vi "Parsing Error (inlined).vi"(7 "JSON":string, 8 "error in (no error)":errorcluster, 9 "Offset past match":i32=-1, 10 "Value start":i32=-1, 11 "State":T1) -> (0 "error out":errorcluster, 3 "Value (if no error)":string)   [LabVIEW 2019, in "JSONtext.lvlib"]
uses:
  JSONtext.lvlib
  Parsing State.ctl
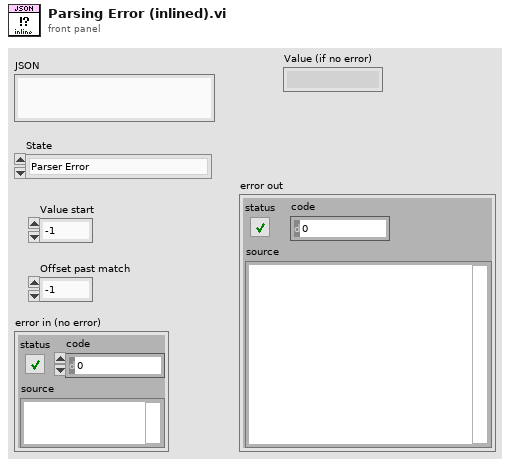
[diagram p1: front panel]
types:
  T1 = typedef "JSONtext.lvlib/Parsing State.ctl" = enum16{"Parser Error", "Object", "Array", "String", "Number/Other", "Leading Whitespace", "Object end", "Array end", "Value end"}
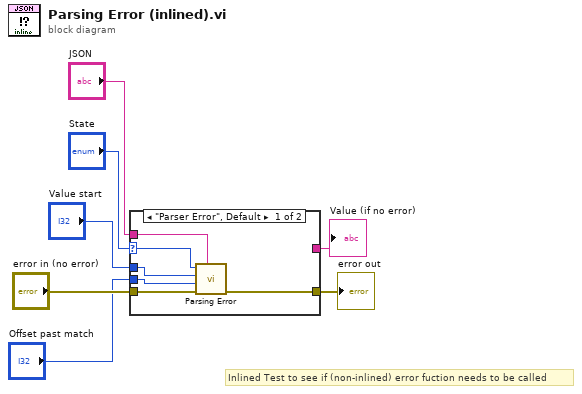
[diagram p0: block diagram]
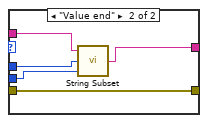
[diagram p2: hidden frame]
diagram:
  # "Inlined Test to see if (non-inlined) error fuction needs to be called"
  n1 = case shown="\"Parser Error\", Default" "State" {
    selector: "State" -> [w8 _]
    tunnel: "JSON" -> [w13 w17]
    tunnel: "error in (no error)" -> [w12 w18]
    tunnel: [w11 w18] -> w6
    tunnel: "Value start" -> [w10 w16]
    tunnel: "Offset past match" -> [w9 w15]
    tunnel: [_ w14] -> w1
    frame "Parser Error", Default {
      n2 = call "Parsing Error.vi"("JSON"=w13, "error in (no error)"=w12, "Offset past match"=w9, "Value start"=w10, "State"=w8) -> ("error out"=w11:errorcluster)  [unwired: 6 in]
    }
    frame "Value end" {
      n3 = call "String Subset.vi"("Offset past End"=w15, "Start offset"=w16, "JSON"=w17) -> ("substring"=w14:string)  [unwired: 2 in]
    }
  }
  "error out" <- w6
  "Value (if no error)" <- w1
